vi "Vary Frequency Continuous with Disc Waveform.vi"() -> ()   [LabVIEW 2020]
uses:
  <vilib>/DAQmx/write.llb/DAQmx Write (Analog Wfm 1Chan NSamp).vi
  <vilib>/DAQmx/create/channels.llb/DAQmx Create Channel (AO-Voltage-Basic).vi
  <vilib>/DAQmx/configure/timing.llb/DAQmx Timing (Use Waveform).vi
  <vilib>/DAQmx/miscellaneous.llb/DAQmx Fill In Error Info.vi
  <vilib>/measure/NI_MABase.lvlib
panel:
  out "Waveform Chart":waveform(dbl)(graph)
  in  "DAQmx Physical Channel":tag
  in  "Blocking Waveform Selection":T1(tab)
  in  "Waveform Type":T2(ring)
  in  "Full Pulse\nWidth (us)":dbl=10.0 min=10.0 step=2.0
  in  "stop":bool
  in  "Waveform\nAmplitude (mAp)":dbl
  in  "Waveform\nFrequency (Hz)":i64=1 min=1 max=100000 step=1
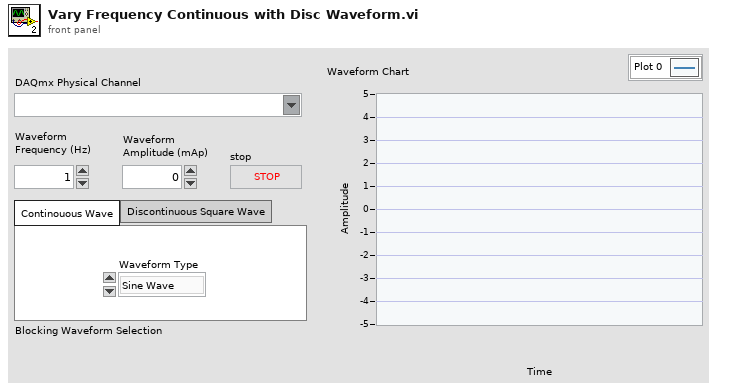
[diagram p1: front panel]
types:
  T1 = enum32{"Continouous Wave", "Discontinuous Square Wave"}
  T2 = enum16{"Sine Wave", "Triangle Wave", "Square Wave", "Sawtooth Wave"}
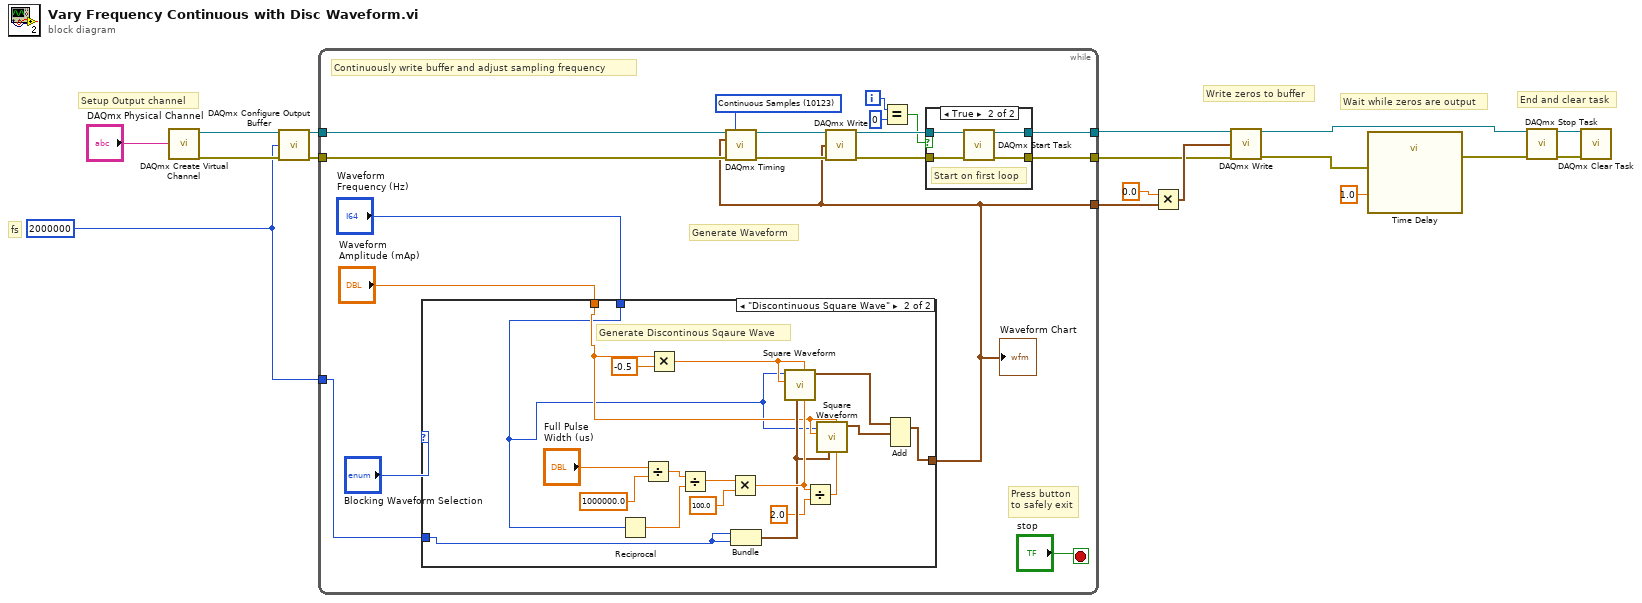
[diagram p0: block diagram]
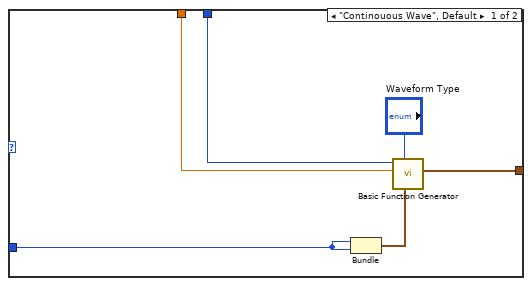
[diagram p2: hidden frame]
diagram:
  w2 = 2000000
  # "fs"
  # "End and clear task"
  # "Wait while zeros are output"
  # "Write zeros to buffer"
  # "Setup Output channel"
  n1 = call-poly <vilib>:"DAQmx Create Virtual Channel.vi"("physical channels"="DAQmx Physical Channel") -> ("task out"=w16:refnum<k21>, "error out"=w17:errorcluster)  [unwired: 13 in]
  n2 = call <vilib>:"DAQmx Configure Output Buffer.vi"("task/channels in"=w16, "buffer size (in samples per channel)"=w2, "error in"=w17) -> ("task out"=w15:refnum<k21>, "error out"=w14:errorcluster)  [unwired: 11 in]
  n3 = while {
    tunnel: w15 -> [w35]
    tunnel: w14 -> [w34]
    tunnel: w2 -> [w20]
    tunnel: [w29] -> w6
    tunnel: [w18] -> w9
    tunnel: [w23] -> w5
    i -> [w25]
    stop <- "stop" stop-if-true
    w27 = 10123 items=["Finite Samples"=10178, "Continuous Samples"=10123, "Hardware Timed Single Point"=12522] ("sample mode")
    # "Press button\nto safely exit"
    # "Generate Waveform"
    # "Continuously write buffer and adjust sampling frequency"
    n4 = case shown="\"Discontinuous Square Wave\"" "Blocking Waveform Selection" {
      tunnel: "Waveform\nFrequency (Hz)" -> [w38 w44]
      tunnel: w20 -> [w37 w43]
      tunnel: "Waveform\nAmplitude (mAp)" -> [w39 w45]
      tunnel: [w36 w42] -> w18
      frame "Continouous Wave", Default {
        n5 = Bundle(w37, w37) -> (w41:cluster{i32, i32})  [unwired: 1 in]
        n6 = call <vilib>:"Basic Function Generator.vi"("sampling info"=w41, "signal type"="Waveform Type", "amplitude"=w39, "frequency"=w38) -> ("signal out"=w36:waveform(dbl))  [unwired: 5 in, 2 out]
      }
      frame "Discontinuous Square Wave" {
        # "Generate Discontinous Sqaure Wave"
        n7 = Reciprocal(x=w44) -> (1/x=w55:dbl)
        n8 = Divide(x="Full Pulse\nWidth (us)", y=1000000.0) -> (x/y=w57:dbl)
        n9 = Multiply(x=w45, y=-0.5) -> (x*y=w52:dbl)
        n10 = Divide(x=w57, y=w55) -> (x/y=w59:dbl)
        n11 = Multiply(x=w59, y=100.0) -> (x*y=w58:dbl)
        n12 = Bundle(w43, w43) -> (w54:cluster{i32, i32})  [unwired: 1 in]
        n13 = call <vilib>:"Square Waveform.vi"("duty cycle (%)"=w58, "offset"=w52, "sampling info"=w54, "amplitude"=w52, "frequency"=w44) -> ("signal out"=w50:waveform(dbl))  [unwired: 5 in, 1 out]
        n14 = Divide(x=w58, y=2.0) -> (x/y=w53:dbl)
        n15 = call <vilib>:"Square Waveform.vi"("duty cycle (%)"=w53, "offset"=w45, "sampling info"=w54, "amplitude"=w45, "frequency"=w44) -> ("signal out"=w51:waveform(dbl))  [unwired: 5 in, 1 out]
        n16 = Add(1:w51, 2:w50) -> (0:w42:waveform(dbl))  [unwired: 1 in, 1 out]
      }
    }
    "Waveform Chart" <- w18
    n17 = call-poly <vilib>:"DAQmx Timing.vi"("task/channels in"=w35, "sample mode"=w27, "waveform"=w18, "error in"=w34) -> ("task out"=w33:refnum<k21>, "error out"=w32:errorcluster)  [unwired: 10 in]
    n18 = call-poly <vilib>:"DAQmx Write.vi"("task/channels in"=w33, "data"=w18, "error in"=w32) -> ("task out"=w31:refnum<k21>, "error out"=w30:errorcluster)  [unwired: 10 in, 1 out]
    n19 = Equal?(x=w25, y=0) -> (x = y?=w26:bool)
    n20 = case shown="True" w26 {
      tunnel: w31 -> [w61 w65]
      tunnel: w30 -> [w60 w64]
      tunnel: [w61 w63] -> w29
      tunnel: [w60 w62] -> w23
      frame False {
      }
      frame True {
        # "Start on first loop"
        n21 = call <vilib>:"DAQmx Start Task.vi"("task/channels in"=w65, "error in"=w64) -> ("task out"=w63:refnum<k21>, "error out"=w62:errorcluster)  [unwired: 12 in]
      }
    }
  }
  n22 = Multiply(x=0.0, y=w9) -> (x*y=w7:waveform(dbl))
  n23 = call-poly <vilib>:"DAQmx Write.vi"("task/channels in"=w6, "data"=w7, "error in"=w5) -> ("task out"=w8:refnum<k21>, "error out"=w4:errorcluster)  [unwired: 10 in, 1 out]
  n24 = call "Time Delay"("error in (no error)"=w4, "Delay Time (s)"=1.0) -> ("error out"=w3:errorcluster)  [unwired: 9 in]
  n25 = call <vilib>:"DAQmx Stop Task.vi"("task/channels in"=w8, "error in"=w3) -> ("task out"=w13:refnum<k21>, "error out"=w12:errorcluster)  [unwired: 12 in]
  n26 = call <vilib>:"DAQmx Clear Task.vi"("task in"=w13, "error in"=w12) -> ()  [unwired: 13 in, 1 out]
